vi "SUB_WrteSFCS_INFO.vi"(2 "Pass/Fail":string) -> ()   [LabVIEW 2011]
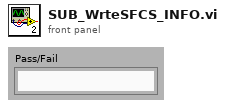
[diagram p1: front panel]
types:
  T1 = enum32{"invalid app kind", "Development System", "Run Time System", "Student Edition", "Embedded LabVIEW", "Evaluation", "Custom"}
  T2 = enum16{"open", "replace", "create", "open or create", "replace or create", "replace or create with confirmation"}
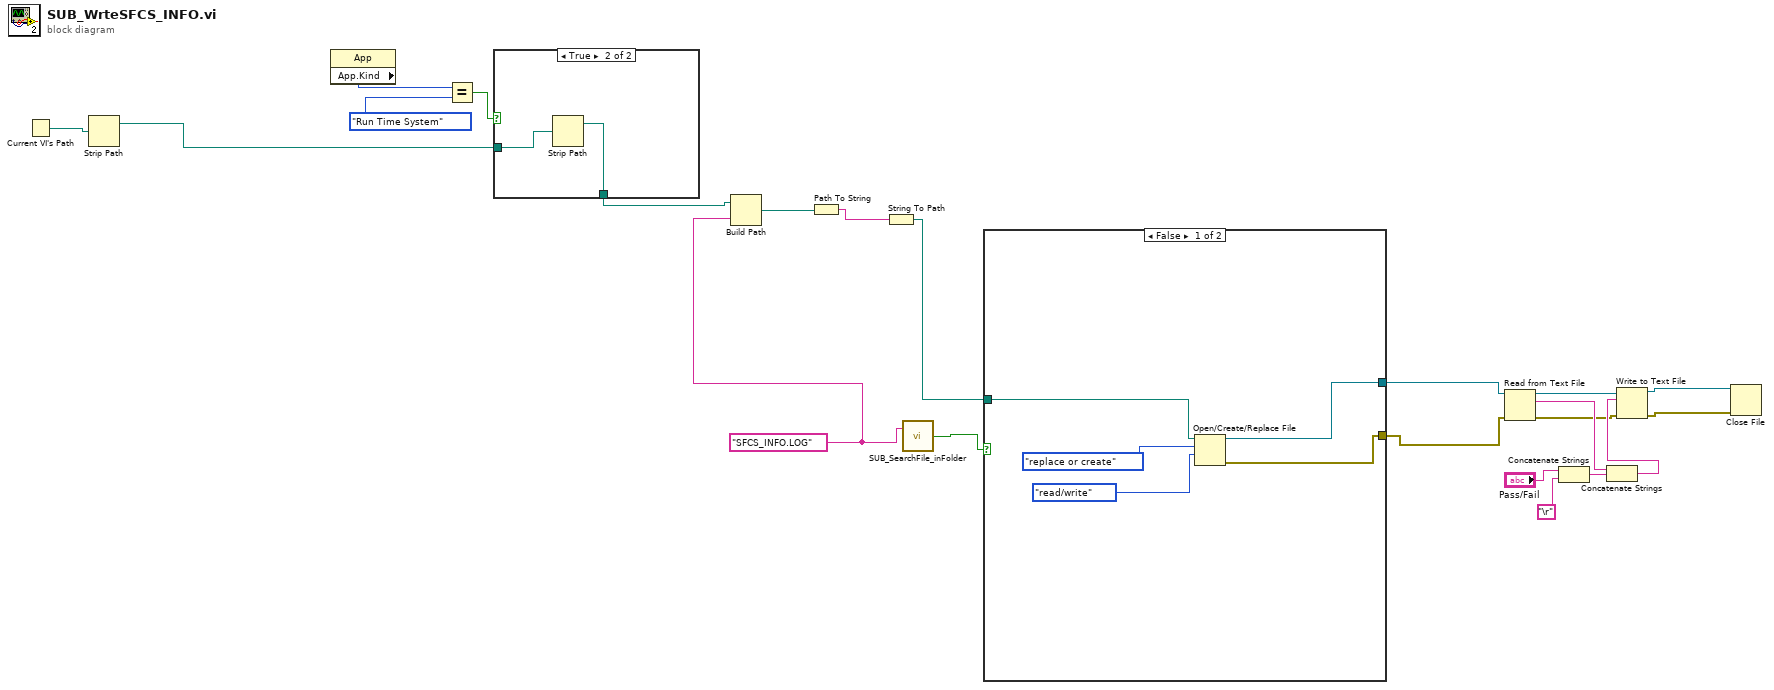
[diagram p0: block diagram]
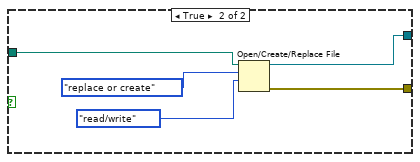
[diagram p2: hidden frame]
diagram:
  w4 = "SFCS_INFO.LOG" ("string")
  n1 = Current VI's Path() -> (path=w18:path)
  n2 = Strip Path(path=w18) -> (stripped path=w14:path)  [unwired: 1 out]
  n3 = property class="App"() -> ("App.Kind"=w17:T1)  [unwired: 2 in, 2 out]
  n4 = Equal?(x=w17, y=T1."Run Time System" ("Application:Kind")) -> (x = y?=w15:bool)
  n5 = case shown="True" w15 {
    tunnel: w14 -> [w23 w25]
    tunnel: [w23 w24] -> w12
    frame False {
    }
    frame True {
      n6 = Strip Path(path=w25) -> (stripped path=w24:path)  [unwired: 1 out]
    }
  }
  n7 = Build Path(base path=w12, name or relative path=w4) -> (appended path=w13:path)
  n8 = Path To String(path=w13) -> (string=w11:string)
  n9 = String To Path(string=w11) -> (path=w3:path)
  n10 = call "SUB_SearchFile_inFolder.vi"("Search Filename in Folder"=w4) -> ("File Existing True/Flase"=w5:bool)  [unwired: 1 in]
  n11 = case shown="False" w5 {
    tunnel: w3 -> [w28 w33]
    tunnel: [w26 w32] -> w2
    tunnel: [w27 w31] -> w1
    frame False {
      n12 = Open/Create/Replace File(file path (use dialog)=w28, operation (0:open)=T2."replace or create", access (0:read/write)=enum16{"read/write", "read-only", "write-only"}."read/write") -> (refnum out=w27:refnum<file>, error out=w26:errorcluster)  [unwired: 3 in, 1 out]
    }
    frame True {
      n13 = Open/Create/Replace File(file path (use dialog)=w33, operation (0:open)=T2."replace or create", access (0:read/write)=enum16{"read/write", "read-only", "write-only"}."read/write") -> (refnum out=w31:refnum<file>, error out=w32:errorcluster)  [unwired: 3 in, 1 out]
    }
  }
  n14 = Read from Text File(file (use dialog)=w1, error in=w2) -> (refnum out=w6:refnum<file>, text=w10:string, error out=w7:errorcluster)  [unwired: 2 in, 1 out]
  n15 = Concatenate Strings("Pass/Fail", "\r") -> (w9:string)
  n16 = Concatenate Strings(w10, w9) -> (w8:string)
  n17 = Write to Text File(file (use dialog)=w6, text=w8, error in=w7) -> (refnum out=w20:refnum<file>, error out=w21:errorcluster)  [unwired: 1 in, 1 out]
  n18 = Close File(refnum=w20, error in=w21) -> ()  [unwired: 2 out]
